vi "Set frequency.vi"(7 "Ignore out of range error (false)":bool, 8 "error in":errorcluster, 10 "Frequency":dbl, 11 "VISA resource name":refnum<visa-resource-name>) -> (0 "error out":errorcluster, 2 "Set frequency failed":bool, 3 "VISA resource name out":refnum<visa-resource-name>)   [LabVIEW 2020, in "Datron D4xxx.lvlib"]
doc: "This VI sets calibrator output frequnecy in AC modes. Optionally you can configure this VI to ignore possible error reported by instrument."
uses:
  Datron D4xxx.lvlib
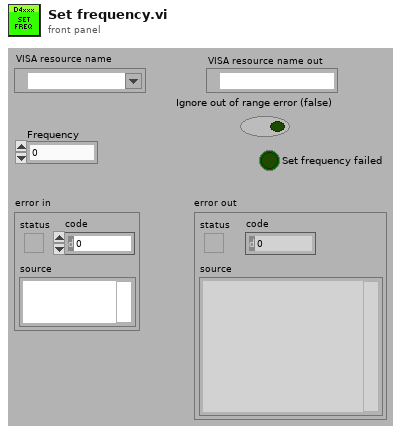
[diagram p1: front panel]
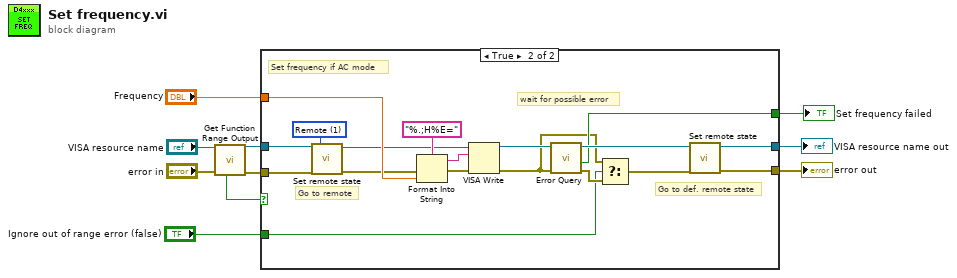
[diagram p0: block diagram]
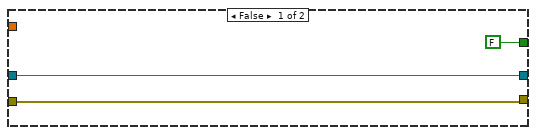
[diagram p2: hidden frame]
diagram:
  n1 = call "Get Function Range Output.vi"("error in (no error)"="error in", "VISA resource name"="VISA resource name") -> ("error out"=w5:errorcluster, "VISA resource name out"=w4:refnum<visa-resource-name>, "AC"=w3:bool)  [unwired: 2 in, 5 out]
  n2 = case shown="True" w3 {
    tunnel: "Frequency" -> [_ w25]
    tunnel: [w13 w28] -> w9
    tunnel: [w12 w27] -> w8
    tunnel: w5 -> [w13 w24]
    tunnel: w4 -> [w12 w23]
    tunnel: [FALSE ("Error") w18] -> w2
    tunnel: "Ignore out of range error (false)" -> [_ w14]
    frame False {
    }
    frame True {
      w20 = u16 1 items=["Local", "Remote", "Default"] ("Remote state")
      # "Go to def. remote state"
      # "Go to remote"
      # "Set frequency if AC mode"
      # "wait for possible error"
      n3 = call "Set remote state.vi"("error in"=w24, "Remote state"=w20, "VISA resource name"=w23) -> ("error out"=w22:errorcluster, "VISA resource name out"=w21:refnum<visa-resource-name>)  [unwired: 7 in]
      n4 = Format Into String(format string="%.;H%E=", error in=w22, w25) -> (resulting string=w31:string, error out=w30:errorcluster)  [unwired: 1 in]
      n5 = VISA Write(VISA resource name=w21, write buffer=w31, error in (no error)=w30) -> (VISA resource name out=w19:refnum<visa-resource-name>, error out=w16:errorcluster)  [unwired: 1 out]
      n6 = call "Error Query.vi"("error in (no error)"=w16, "VISA resource name"=w19) -> ("error out"=w17:errorcluster, "Error"=w18:bool, "VISA resource name out"=w26:refnum<visa-resource-name>)  [unwired: 6 in, 1 out]
      n7 = Select(t=w16, s=w14, f=w17) -> (s? t:f=w15:errorcluster)
      n8 = call "Set remote state.vi"("error in"=w15, "VISA resource name"=w26) -> ("error out"=w28:errorcluster, "VISA resource name out"=w27:refnum<visa-resource-name>)  [unwired: 8 in]
    }
  }
  "VISA resource name out" <- w8
  "error out" <- w9
  "Set frequency failed" <- w2
